vi "Change Screen.vi"(8 "error in (no error)":errorcluster, 10 "Screen":string, 11 "Assert Display in":refnum<class "Assert Display.lvclass">) -> (0 "error out":errorcluster, 3 "Assert Display out":refnum<class "Assert Display.lvclass">)   [LabVIEW 2016, in "Assert Display.lvlib" / "Assert Display.lvclass"]
doc: "Sends a message to the appropriate screen to insert itself into the main UI subpanel"
uses:
  Assert Display.lvclass
  Assert Display.lvclass/Assert Display.ctl
  <vilib>/ActorFramework/Message Enqueuer/Message Enqueuer.lvclass/Message Enqueuer.ctl
  <vilib>/ActorFramework/Message Enqueuer/Enqueue.vi
  Base UI Component/Base UI Component Messages/Insert to Screen Msg/Insert to Screen Msg.lvclass
  C:/Program Files (x86)/National Instruments/LabVIEW 2016/vi.lib/ActorFramework/Message/Message.lvclass
  <vilib>/ActorFramework/Message Priority Queue/Priority Enqueue.vi
  <vilib>/ActorFramework/Message Enqueuer/Message Enqueuer.lvclass
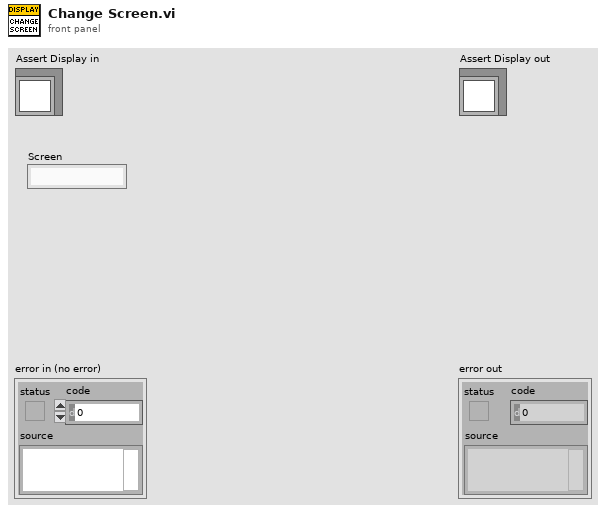
[diagram p1: front panel]
types:
  T1 = cluster{"Main Screen":refnum<class "Message Enqueuer.lvclass">, "Services Screen":refnum<class "Message Enqueuer.lvclass">, "Filters Screen":refnum<class "Message Enqueuer.lvclass">}
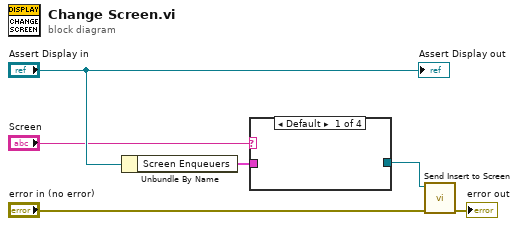
[diagram p0: block diagram]
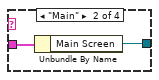
[diagram p2: hidden frame]
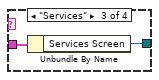
[diagram p3: hidden frame]
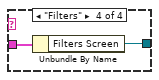
[diagram p4: hidden frame]
diagram:
  n1 = Unbundle By Name("Assert Display in") -> ("Screen Enqueuers"=w4:T1)
  n2 = case shown="Default" "Screen" {
    tunnel: w4 -> [_ w8 w10 w12]
    tunnel: [_ w7 w9 w11] -> w1
    frame Default {
    }
    frame "Main" {
      n3 = Unbundle By Name(w8) -> ("Main Screen"=w7:refnum<class "Message Enqueuer.lvclass">)
    }
    frame "Services" {
      n4 = Unbundle By Name(w10) -> ("Services Screen"=w9:refnum<class "Message Enqueuer.lvclass">)
    }
    frame "Filters" {
      n5 = Unbundle By Name(w12) -> ("Filters Screen"=w11:refnum<class "Message Enqueuer.lvclass">)
    }
  }
  n6 = call "Send Insert to Screen.vi"("error in (no error)"="error in (no error)", "Message Enqueuer"=w1) -> ("error out"=→"error out":errorcluster)  [unwired: 8 in, 1 out]
  "Assert Display out" <- "Assert Display in"
